vi "VISA Recover.vi"(8 "Error In":errorcluster, 11 "VISA resource name":refnum<visa-resource-name>) -> (0 "Error Out":errorcluster, 3 "VISA resource name out":refnum<visa-resource-name>)   [LabVIEW 2021]
uses:
  f46bd5af-de24-4e9e-a8e8-95635435b45a.vi
  <vilib>/Utility/error.llb/Clear Errors.vi
  <vilib>/Utility/error.llb/Error Cluster From Error Code.vi
  <vilib>/ErrorRing/Error Ring.xnode
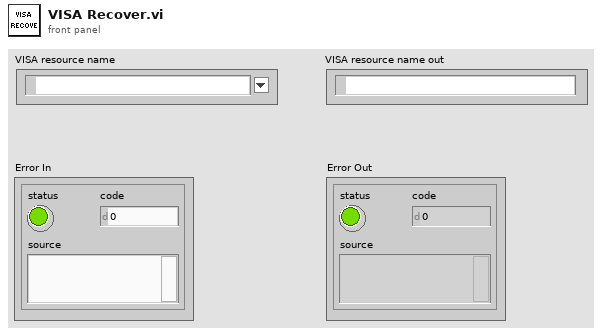
[diagram p1: front panel]
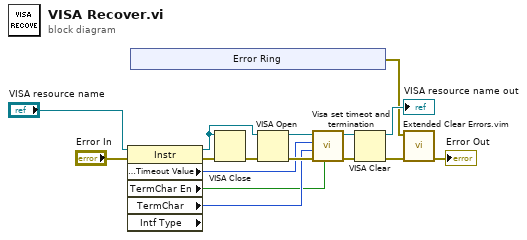
[diagram p0: block diagram]
diagram:
  n1 = property class="Instr" props=["General Settings:Timeout Value", "TermChar En", "TermChar", "Intf Type"](reference="VISA resource name", error in="Error In") -> (reference out=w7:refnum<visa-resource-name>, error out=w5:errorcluster, "General Settings:Timeout Value"=w2:u32, "TermChar En"=w1:bool, "TermChar"=w3:u8)  [unwired: 1 out]
  n2 = xnode "Error Ring"() -> ("error out"=w10:errorcluster)
  n3 = VISA Close(VISA resource name=w7, error in (no error)=w5) -> (error out=w4:errorcluster)
  n4 = VISA Open(error in (no error)=w4, VISA resource name=w7) -> (VISA resource name=w14:refnum<visa-resource-name>, error out=w12:errorcluster)  [unwired: 3 in]
  n5 = call "Visa set timeot and termination.vi"("Termination Character Enable"=w1, "error in (no error)"=w12, "Termination Character"=w3, "Timeout Value"=w2, "VISA resource name"=w14) -> ("error out"=w13:errorcluster, "VISA resource name out"=w8:refnum<visa-resource-name>)  [unwired: 2 in, 3 out]
  n6 = VISA Clear(VISA resource name=w8, error in (no error)=w13) -> (VISA resource name out=→"VISA resource name out":refnum<visa-resource-name>, error out=w15:errorcluster)
  n7 = call "Extended Clear Errors.vim"("Error In"=w15, "specific error code to clear (0: all)"=w10) -> ("Error Out"=→"Error Out":errorcluster)  [unwired: 7 in, 2 out]
